vi "Set Temperature.vi"(8 "error in (no error)":errorcluster, 10 "Setpoint":dbl, 11 "Julabo Fp-50 Settings":T1={"VISA resource name"="", "Simulated?"=FALSE, "Pump Power"=2} {"Pump Power" min=0 max=8 step=1}) -> (0 "error out":errorcluster, 1 "Connection Error":bool, 3 "Julabo FP-50 Settings":T1={"VISA resource name"="", "Simulated?"=FALSE, "Pump Power"=2} {"Pump Power" min=0 max=8 step=1})   [LabVIEW 2018, in "Julabo Type FP-50 TCU.lvlib"]
uses:
  Julabo Type FP-50 TCU.lvlib
  Julabo FP-50 Settings.ctl
  Third Party Drivers/Julabo Type 1/JULABO DeviceDriver/JULABO DeviceDriver.lvlib
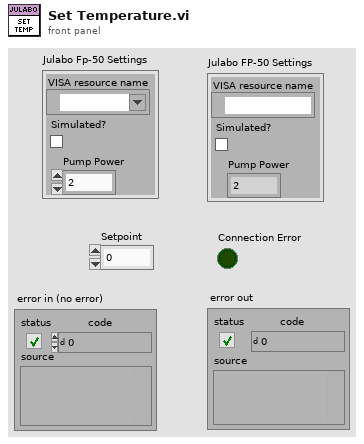
[diagram p1: front panel]
types:
  T1 = typedef "Julabo Type FP-50 TCU.lvlib/Julabo FP-50 Settings.ctl" = cluster{"VISA resource name":refnum<visa-resource-name>, "Simulated?":bool, "Pump Power":i32}
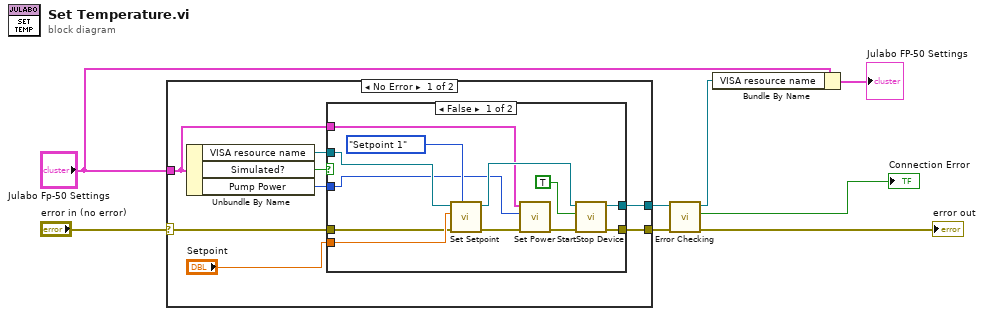
[diagram p0: block diagram]
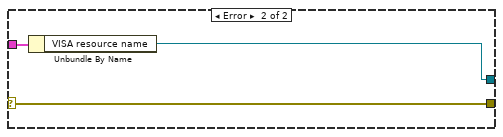
[diagram p3: hidden frame]
diagram:
  n1 = case shown="No Error" "error in (no error)" {
    selector: "error in (no error)" -> [w16 w33]
    tunnel: "Julabo Fp-50 Settings" -> [w11 w32]
    tunnel: [w15 w33] -> w6
    tunnel: [w13 w31] -> w7
    frame No Error {
      n2 = Unbundle By Name(w11) -> ("VISA resource name"=w14:refnum<visa-resource-name>, "Simulated?"=w12:bool, "Pump Power"=w9:i32)
      n3 = case shown="False" w12 {
        tunnel: w16 -> [w23 w30]
        tunnel: [w17 w30] -> w15
        tunnel: [w22 w29] -> w13
        tunnel: w14 -> [w25 w29]
        tunnel: w11 -> [w21 _]
        tunnel: "Setpoint" -> [w28 _]
        tunnel: w9 -> [w20 _]
        frame False {
          n4 = call "Set Setpoint.vi"("Setpointindex (Setpoint1: Default)"=enum16{"Setpoint 1", "Setpoint 2", "Setpoint 3"}."Setpoint 1", "error in (no error)"=w23, "newSetpoint (20.00°C)"=w28, "VISA resource name"=w25) -> ("error out"=w19:errorcluster, "VISA resource name out"=w24:refnum<visa-resource-name>)  [unwired: 6 in]
          n5 = call "Set Power.vi"("error in (no error)"=w19, "Power"=w20, "Julabo FP-50 Settings"=w21) -> ("error out"=w18:errorcluster)  [unwired: 6 in, 2 out]
          n6 = call "StartStop Device.vi"("error in (no error)"=w18, "Start/Stop (f:Stop)"=TRUE, "VISA resource name"=w24) -> ("error out"=w17:errorcluster, "VISA resource name out"=w22:refnum<visa-resource-name>)  [unwired: 7 in]
        }
        frame True {
        }
      }
    }
    frame Error {
      n7 = Unbundle By Name(w32) -> ("VISA resource name"=w31:refnum<visa-resource-name>)
    }
  }
  n8 = call "Error Checking.vi"("error in (no error)"=w6, "VISA resource name"=w7) -> ("error out"=→"error out":errorcluster, "Connection Error"=→"Connection Error":bool, "VISA resource name"=w4:refnum<visa-resource-name>)  [unwired: 7 in]
  n9 = Bundle By Name(cluster="Julabo Fp-50 Settings", "VISA resource name"=w4) -> (→"Julabo FP-50 Settings":T1)
